vi "niTuner Set Attenuation.vi"(8 "error in":errorcluster, 9 "mixer level (dBm)":i32=-20, 10 "ref level (dBm)":i32, 11 "taskID in":i32 format="%.0x") -> (0 "error out":errorcluster, 1 "scale factor":dbl format="%.2f", 2 "attenuation":dbl format="%.2f", 3 "taskID out":i32 format="%.0x")   [LabVIEW 2011]
doc: "This VI sets the PXI-5600 internal attenuators based upon your <B>reference level</B> and <B>mixer level</B> settings.\n\n<B>NOTE:</B> If new center frequencies of less than 15 MHz are specified after a call to this VI, attenuation may be automatically adjusted. Up to 20 dB of additional attenuation may be added."
uses:
  nipxi5600u.dll
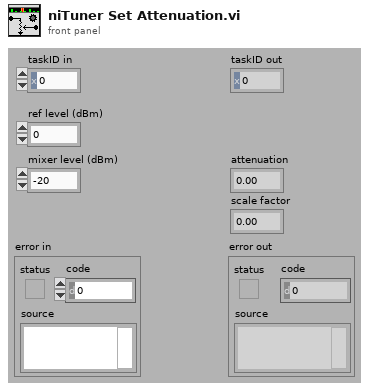
[diagram p1: front panel]
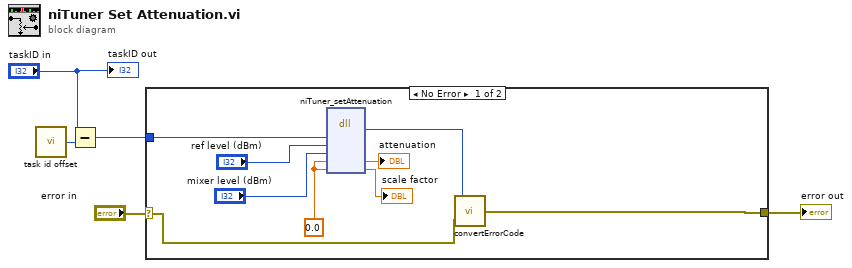
[diagram p0: block diagram]
diagram:
  n1 = call <instrlib>:"task id offset.vi"() -> ("taskID offset"=w2:i32)
  n2 = Subtract(x="taskID in", y=w2) -> (x-y=w3:i32)
  n3 = case shown="No Error" "error in" {
    selector: "error in" -> [w7 w15]
    tunnel: [w6 w15] -> w4
    tunnel: w3 -> [w14 _]
    frame No Error {
      w13 = 0.0
      n4 = dll-call lib="nipxi5600u.dll" fn="niTuner_setAttenuation"("taskID"=w14, "refLevel"="ref level (dBm)", "mixerLevel"="mixer level (dBm)", "attenuation"=w13, "scaleFactor"=w13) -> (w8:i32, "attenuation"=→"attenuation":dbl, "scaleFactor"=→"scale factor":dbl)  [unwired: 6 in, 2 out]
      n5 = call <instrlib>:"convertErrorCode.vi"("error in"=w7, "error code"=w8) -> ("error out"=w6:errorcluster)
    }
    frame Error {
    }
  }
  "error out" <- w4
  "taskID out" <- "taskID in"
